vi "BIN_FileRef_Split_Header_and_content.vi"(8 "error in":errorcluster, 11 "refnum in":refnum<file>) -> (0 "error out":errorcluster, 1 "Content":string, 2 "TAGs":string[](array[string]), 3 "refnum out":refnum<file>, 5 "start of data":i64)   [LabVIEW 2020, in "DBAL-BIN.lvclass"]
doc: "Read header file portion of Historian Database file,\nbased on a file reference, and keep file open."
uses:
  DBAL-BIN.lvclass
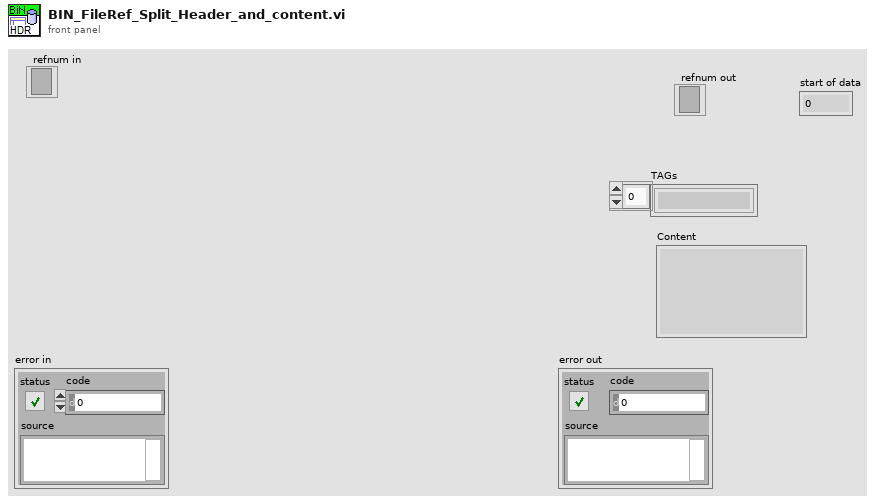
[diagram p1: front panel]
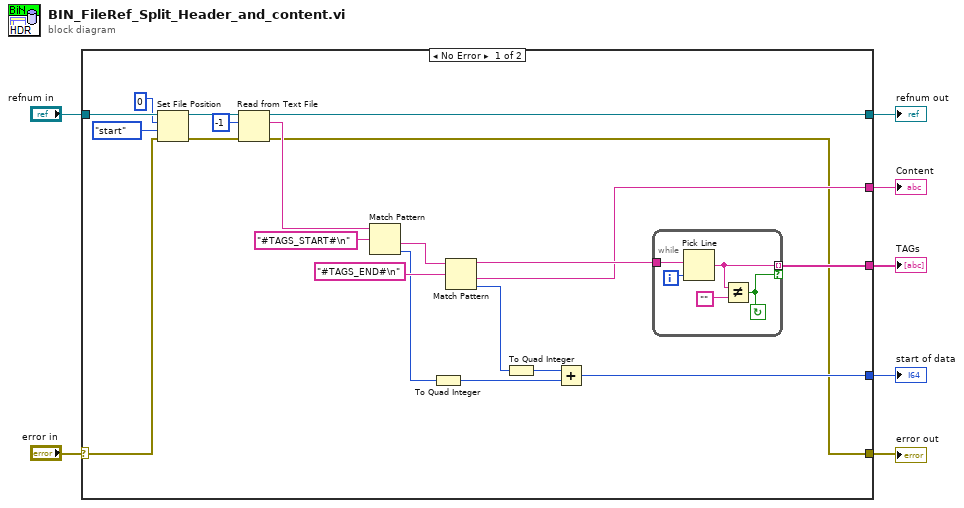
[diagram p0: block diagram]
diagram:
  n1 = case shown="No Error" "error in" {
    selector: "error in" -> [w11 w35]
    tunnel: [w17 w35] -> w6
    tunnel: "refnum in" -> [w12 w34]
    tunnel: [w16 w34] -> w1
    tunnel: [w23 _] -> w5
    tunnel: [w22 _] -> w4
    tunnel: [w18 _] -> w3
    frame No Error {
      n2 = Set File Position(offset (in bytes) (0)=i64 0, refnum=w12, from (0:start)=enum16{"start", "end", "current"}."start", error in=w11) -> (refnum out=w13:refnum<file>, error out=w10:errorcluster)
      n3 = Read from Text File(file (use dialog)=w13, count=-1, error in=w10) -> (refnum out=w16:refnum<file>, text=w28:string, error out=w17:errorcluster)  [unwired: 1 in, 1 out]
      n4 = Match Pattern(string=w28, regular expression="#TAGS_START#\n") -> (after substring=w26:string, offset past match=w20:i32)  [unwired: 1 in, 2 out]
      n5 = To Quad Integer(1:w20) -> (0:w14:i64)
      n6 = Match Pattern(string=w26, regular expression="#TAGS_END#\n") -> (before substring=w24:string, after substring=w22:string, offset past match=w21:i32)  [unwired: 1 in, 1 out]
      n7 = To Quad Integer(1:w21) -> (0:w15:i64)
      n8 = Add(x=w15, y=w14) -> (x+y=w18:i64)
      n9 = while {
        tunnel: w24 -> [w29]
        tunnel: [w32] -> w23 mode=indexing if=w30
        i -> [w33]
        stop <- w30 continue-if-true
        n10 = Pick Line(multi-line string=w29, line index=w33) -> (output string=w32:string)  [unwired: 1 in]
        n11 = Not Equal?(x=w32, y="") -> (x != y?=w30:bool)
      }
    }
    frame Error {
    }
  }
  "error out" <- w6
  "TAGs" <- w5
  "Content" <- w4
  "start of data" <- w3
  "refnum out" <- w1
